vi "Line Detection.vi"   [LabVIEW 2018]
uses:
  <vilib>/Rock Robotics/WPI/Utilities/WPI_GetSetVariantRefNum.vi
  Drive Published Globals.vi
  <vilib>/ptbypt/NI_PtbyPt.lvlib
types:
  T1 = typedef "WPI_SwitchDevRef.ctl" = cluster{"DevStatus":errorcluster, "DIO Channel":T2, "CntIndex":T3, "Normally Closed":bool}
  T2 = typedef "FPGA_DIOChannel.ctl" = enum8{"DIO 0", "DIO 1", "DIO 2", "DIO 3", "DIO 4", "DIO 5", "DIO 6", "DIO 7", "DIO 8", "DIO 9", "DIO MXP 0", "DIO MXP 1", "DIO MXP 2", "DIO MXP 3", "DIO MXP 4", "DIO MXP 5", "DIO MXP 6", "DIO MXP 7", "DIO MXP 8", "DIO MXP 9", "DIO MXP 10", "DIO MXP 11", "DIO MXP 12", "DIO MXP 13", "DIO MXP 14", "DIO MXP 15", "SPI Port CS1", "SPI Port CS2", "SPI Port CS3", "SPI Port MISO", "SPI Port MOSI", "Invalid"}
  T3 = typedef "FPGA_CounterCtrSystemIndex.ctl" = enum8{"Ctr 0", "Ctr 1", "Ctr 2", "Ctr 3", "Ctr 4", "Ctr 5", "Ctr 6", "Ctr 7", "Invalid"}
  T4 = typedef "WPI_JoystickDevRef.ctl" = cluster{"Device":T5}
  T5 = typedef "WPI_JoystickDeviceEnum.ctl" = enum16{"USB 0", "USB 1", "USB 2", "USB 3", "USB 4", "USB 5"}
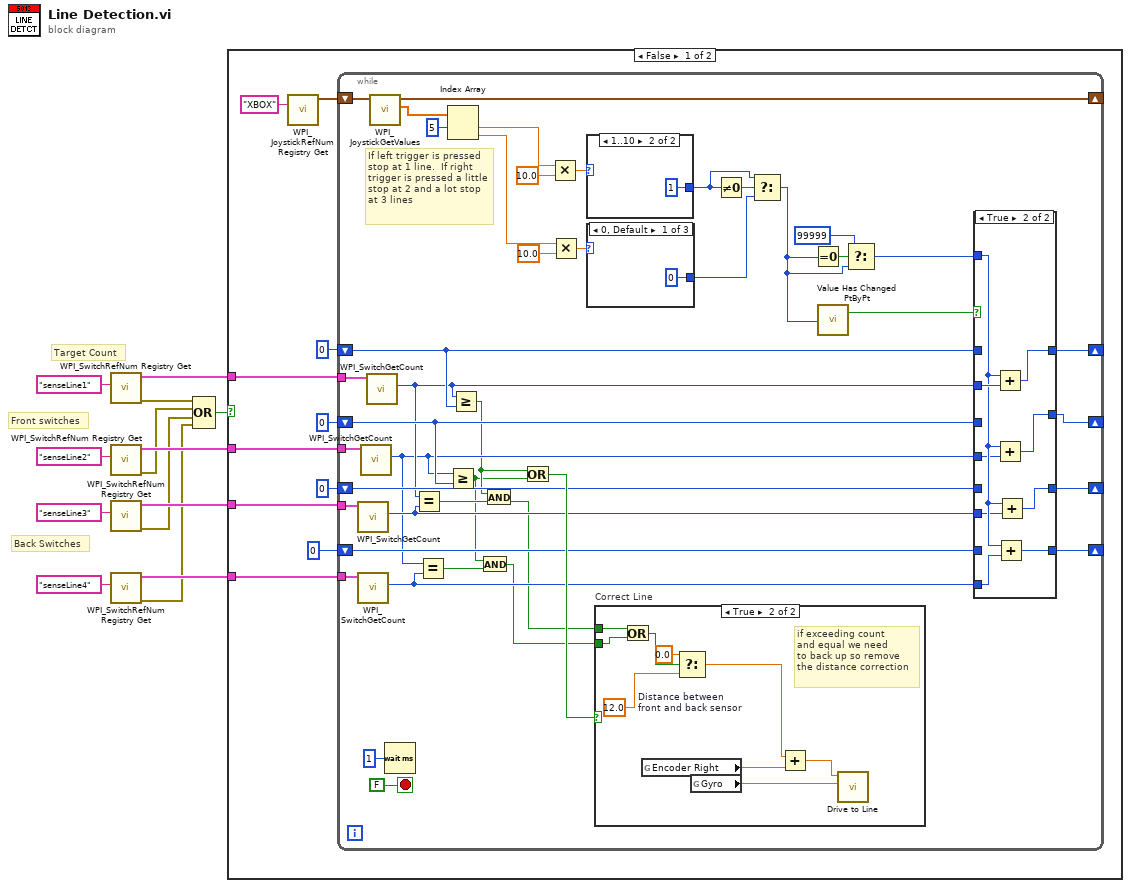
[diagram p0: block diagram]
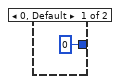
[diagram p3: hidden frame]
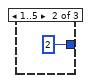
[diagram p4: hidden frame]
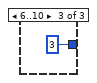
[diagram p5: hidden frame]
diagram:
  # "Back Switches"
  # "Front switches"
  # "Target Count"
  n1 = call <vilib>:"WPI_SwitchRefNum Registry Get.vi"("refnum name"="senseLine1") -> ("error out"=w5:errorcluster, "SwitchDevRef"=w13:T1)  [unwired: 9 in]
  n2 = call <vilib>:"WPI_SwitchRefNum Registry Get.vi"("refnum name"="senseLine2") -> ("error out"=w4:errorcluster, "SwitchDevRef"=w10:T1)  [unwired: 9 in]
  n3 = call <vilib>:"WPI_SwitchRefNum Registry Get.vi"("refnum name"="senseLine3") -> ("error out"=w3:errorcluster, "SwitchDevRef"=w6:T1)  [unwired: 9 in]
  n4 = call <vilib>:"WPI_SwitchRefNum Registry Get.vi"("refnum name"="senseLine4") -> ("error out"=w2:errorcluster, "SwitchDevRef"=w9:T1)  [unwired: 9 in]
  n5 = Compound Arithmetic op=OR(w5, w4, w3, w2) -> (w1:bool)
  n6 = case shown="False" w1 {
    tunnel: w13 -> [w21 _]
    tunnel: w10 -> [w20 _]
    tunnel: w9 -> [w17 _]
    tunnel: w6 -> [w16 _]
    frame False {
      n7 = call <vilib>:"WPI_JoystickRefNum Registry Get.vi"("refnum name"="XBOX") -> ("JoystickDevRef"=w18:T4)  [unwired: 1 in, 9 out]
      n8 = while {
        shift-right: [w63] -> _
        shift-left: w18 -> [w64]
        tunnel: w21 -> [w62]
        shift-right: [w39] -> _
        shift-left: 0 ("length") -> [w40]
        shift-right: [w44] -> _
        shift-left: 0 ("length") -> [w34]
        tunnel: w20 -> [w61]
        tunnel: w16 -> [w41]
        shift-right: [w36] -> _
        shift-left: 0 ("length") -> [w37]
        tunnel: w17 -> [w42]
        shift-right: [w35] -> _
        shift-left: 0 ("length") -> [w38]
        stop <- FALSE stop-if-true
        # "If left trigger is pressed\nstop at 1 line.  If right\ntrigger is pressed a little\nstop at 2 and a lot stop\nat 3 lines"
        n9 = call <vilib>:"WPI_SwitchGetCount.vi"("SwitchDevRef"=w41) -> ("Switch Pressed Count"=w33:i32)  [unwired: 8 in, 2 out]
        n10 = call <vilib>:"WPI_SwitchGetCount.vi"("SwitchDevRef"=w42) -> ("Switch Pressed Count"=w30:i32)  [unwired: 8 in, 2 out]
        n11 = call <vilib>:"WPI_SwitchGetCount.vi"("SwitchDevRef"=w61) -> ("Switch Pressed Count"=w29:i32)  [unwired: 8 in, 2 out]
        n12 = call <vilib>:"WPI_SwitchGetCount.vi"("SwitchDevRef"=w62) -> ("Switch Pressed Count"=w32:i32)  [unwired: 8 in, 2 out]
        n13 = call <vilib>:"WPI_JoystickGetValues.vi"("JoystickDevRef"=w64) -> ("Axes"=w56:dbl[], "JoystickDevRef"=w63:T4)  [unwired: 6 in, 3 out]
        n14 = Wait (ms)(milliseconds to wait=u32 1) -> ()  [unwired: 1 out]
        n15 = Equal?(x=w32, y=w33) -> (x = y?=w31:bool)
        n16 = Equal?(x=w29, y=w30) -> (x = y?=w26:bool)
        n17 = Index Array(array=w56, index #1=5 ("index")) -> (element #1=w54:dbl, element #2=w53:dbl)  [unwired: 1 in]
        n18 = Greater Or Equal?(x=w29, y=w40) -> (x >= y?=w25:bool)
        n19 = Greater Or Equal?(x=w32, y=w34) -> (x >= y?=w27:bool)
        n20 = And(x=w25, y=w26) -> (x .and. y?=w24:bool)
        n21 = And(x=w27, y=w31) -> (x .and. y?=w28:bool)
        n22 = Or(x=w27, y=w25) -> (x .or. y?=w43:bool)
        n23 = Multiply(x=w54, y=10.0) -> (x*y=w59:dbl)
        n24 = Multiply(x=w53, y=10.0) -> (x*y=w60:dbl)
        n25 = case shown="1..10" w59 {
          tunnel: [0 1] -> w51
          frame 0, Default {
          }
          frame 1..10 {
          }
        }
        n26 = case shown="0, Default" w60 {
          tunnel: [0 2 3] -> w50
          frame 0, Default {
          }
          frame 1..5 {
          }
          frame 6..10 {
          }
        }
        n27 = case "Correct Line" shown="True" w43 {
          tunnel: w24 -> [_ w89]
          tunnel: w28 -> [_ w90]
          frame False {
          }
          frame True {
            w88 = 12.0  # Distance between front and back sensor
            # "if exceeding count\nand equal we need\nto back up so remove\nthe distance correction"
            n28 = Or(x=w90, y=w89) -> (x .or. y?=w87:bool)
            n29 = global read "Drive Published Globals.vi" "Encoder Right"() -> (w93:dbl)
            n30 = Select(t=0.0, s=w87, f=w88) -> (s? t:f=w85:dbl)
            n31 = global read "Drive Published Globals.vi" "Gyro"() -> (w91:dbl)
            n32 = Add(x=w85, y=w93) -> (x+y=w92:dbl)
            n33 = call "Drive to Line.vi"("Target Angle"=w91, "Distance"=w92) -> ()  [unwired: 9 in, 1 out]
          }
        }
        n34 = Not Equal To 0?(x=w51) -> (x != 0?=w52:bool)
        n35 = Select(t=w51, s=w52, f=w50) -> (s? t:f=w47:i32)
        n36 = Equal To 0?(x=w47) -> (x = 0?=w48:bool)
        n37 = call <vilib>:"Value Has Changed PtByPt.vi"("input data point"=w47) -> ("has changed"=w49:bool)  [unwired: 1 in, 1 out]
        n38 = Select(t=99999, s=w48, f=w47) -> (s? t:f=w45:i32)
        n39 = case shown="True" w49 {
          tunnel: w32 -> [_ w79]
          tunnel: w45 -> [_ w76]
          tunnel: [w70 w78] -> w44
          tunnel: w40 -> [w69 _]
          tunnel: [w69 w77] -> w39
          tunnel: w38 -> [w68 _]
          tunnel: w37 -> [w67 _]
          tunnel: [w67 w75] -> w36
          tunnel: [w68 w74] -> w35
          tunnel: w34 -> [w70 _]
          tunnel: w29 -> [_ w73]
          tunnel: w33 -> [_ w72]
          tunnel: w30 -> [_ w71]
          frame False {
          }
          frame True {
            n40 = Add(x=w76, y=w79) -> (x+y=w78:i32)
            n41 = Add(x=w76, y=w73) -> (x+y=w77:i32)
            n42 = Add(x=w76, y=w71) -> (x+y=w75:i32)
            n43 = Add(x=w76, y=w72) -> (x+y=w74:i32)
          }
        }
      }
    }
    frame True {
    }
  }
